vi "test_ThreeSessThreePinTwoInstrTwoSiteReservation_CallGetConnectionsFromPinsWithNoMatchingConnections_ReturnsError.vi"(8 "error in":errorcluster) -> (0 "error out":errorcluster, 2 "result":string, 3 "pass":bool)   [LabVIEW 2020, in "MeasurementServerTests.lvlib"]
uses:
  MeasurementServerTests.lvlib
  Runtime/Measurement Plugin Session Management V1/Session Reservation/Connection with Session.ctl
  Runtime/Measurement Plugin Session Management V1/Session Reservation/Connection.ctl
  Runtime/Measurement Plugin Session Management V1/Session Reservation/Pin Type.ctl
  Runtime/MeasurementLink niFGEN/Session Factory/Session Factory.lvclass
  C:/dev/measurementlink-labview/Source/Runtime/MeasurementLink Instrument/ISession Factory/ISession Factory.lvclass
  c3cb69a0-23cd-49fc-99d1-8c54773f0200.vi
  Runtime/Measurement Plugin Session Management V1/Session Reservation/Get Connections Impl.vi
  Runtime/Measurement Plugin Measurement Server/Helpers/Error Strings Global Internal.vi
  Runtime/Measurement Plugin Session Management V1/Session Reservation/Session Reservation.lvclass
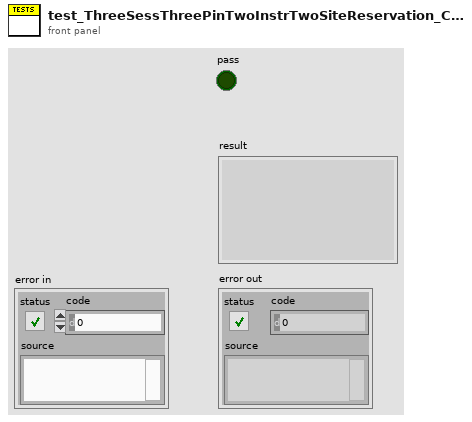
[diagram p1: front panel]
types:
  T1 = typedef "Measurement Plugin Session Management V1.lvlib/Session Reservation.lvclass/Pin Type.ctl" = enum16{"DUT and System Pins", "System Pins"}
  T2 = typedef "Measurement Plugin Session Management V1.lvlib/Session Reservation.lvclass/Connection with Session.ctl" = cluster{"connection":T3, "session":variant}
  T3 = typedef "Measurement Plugin Session Management V1.lvlib/Session Reservation.lvclass/Connection.ctl" = cluster{"pin or relay name":string, "site":i32, "instrument type id":string, "channel":string}
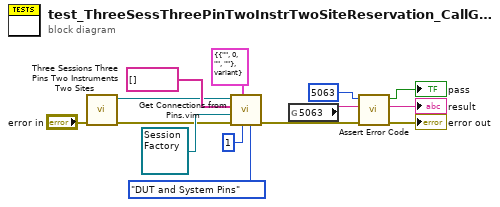
[diagram p0: block diagram]
diagram:
  n1 = call "Three Sessions Three Pins Two Instruments Two Sites.vi"("error in"="error in") -> ("error out"=w2:errorcluster, "session reservation out"=w1:refnum<class "Session Reservation.lvclass">)  [unwired: 8 in, 1 out]
  n2 = call "Get Connections from Pins.vim"("pin type"=Pin_Type."DUT and System Pins", "site"=1, "connection type"=T2 {"connection"={"pin or relay name"="", "site"=0, "instrument type id"="", "channel"=""}, "session"=variant} ("connection"), "error in"=w2, "session factory"=refnum<class "Session Factory.lvclass"> refnum ("MeasurementLink niFGEN.lvlib:Instrument.lvclass"), "pin or relay names"=string[] [], "session reservation in"=w1) -> ("error out"=w9:errorcluster)  [unwired: 2 in, 2 out]
  n3 = global read "Error Strings Global Internal.vi" "5063"() -> (w10:string)
  n4 = call "Assert Error Code.vi"("error in"=w9, "expected error description"=w10, "expected error code"=5063) -> ("error out"=→"error out":errorcluster, "details"=→"result":string, "error code match?"=→"pass":bool)  [unwired: 6 in]
